vi "Spec Edit.vi"(4 "0기준?":bool, 5 "Condition":string[][](table), 6 "열번호(기준값)":i32, 7 "Spec Value":string[][](table), 8 "에러 입력(에러 없음)":errorcluster, 9 "Resolution":string[][](array[string]), 10 "Spec Default":string[][](table), 11 "Func_ext":string) -> (0 "에러 출력":errorcluster, 1 "변경?":bool, 2 "Spec Default out":string[][](array[string]), 3 "Spec 출력":string[][](array[string]))   [LabVIEW 2020]
uses:
  Controls/Cmd_Spec Edit.ctl
  Controls/Cmd_Mouse Popup.ctl
  Controls/Cmd_Var Data IO.ctl
  Variables/Global_Cal Info.vi
  Public/Polymorph/Cell Space_Table.vi
panel:
  in  "추가 단위":string
  in  "추가SPEC":string
  in  "적용":bool
  in  "초기화":bool
  in  "Default 단위":string
  in  "일괄변경":bool
  in  "하한":bool
  in  "상한":bool
  in  "상한하한":bool
  in  "스크롤 막대":i32(c297)
  in  "Default 값":string
  in  "취소":bool
  in  "확인":bool
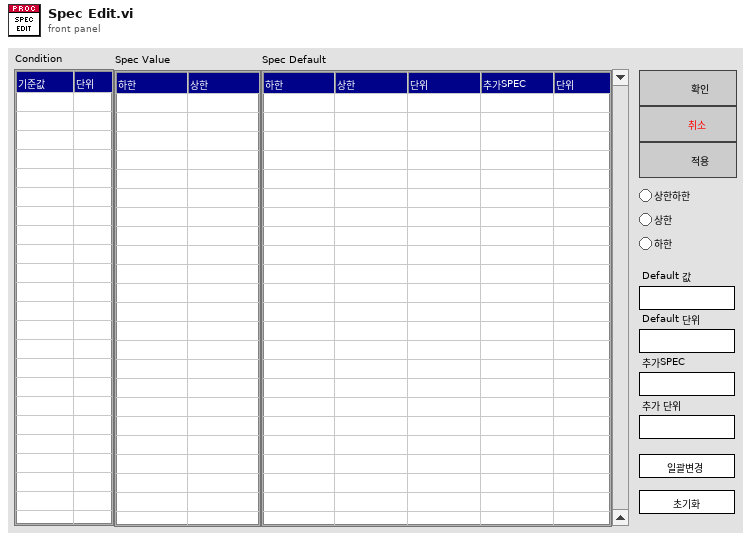
[diagram p1: front panel]
types:
  T1 = typedef "Cmd_Spec Edit.ctl" = enum16{"종료", "Start", "스펙계산", "이벤트대기"}
  T2 = typedef "Cmd_Mouse Popup.ctl" = enum16{"활성화", "메뉴선택"}
  T3 = typedef "Cmd_Var Data IO.ctl" = enum16{"Condition", "Condition Default", "Condition_Temp", "Resolution", "Resolution Default", "Resolution Old", "Spec", "Spec Default", "Spec Old", "Spec Temp", "Result", "Result2", "Result3", "Result_Temp", "Result_ADJ", "Result_ADJ2", "STD1", "STD2", "STD3", "STD4", "STD5", "STD Temp", "CMC", "CMC Default"}
  T4 = typedef "LVRectTypeDef.ctl" = cluster{"Left":i16, "Top":i16, "Right":i16, "Bottom":i16}
  T5 = cluster{"Shift":bool, "Ctrl":bool, "Alt":bool, "Cmd":bool, "Opt":bool}
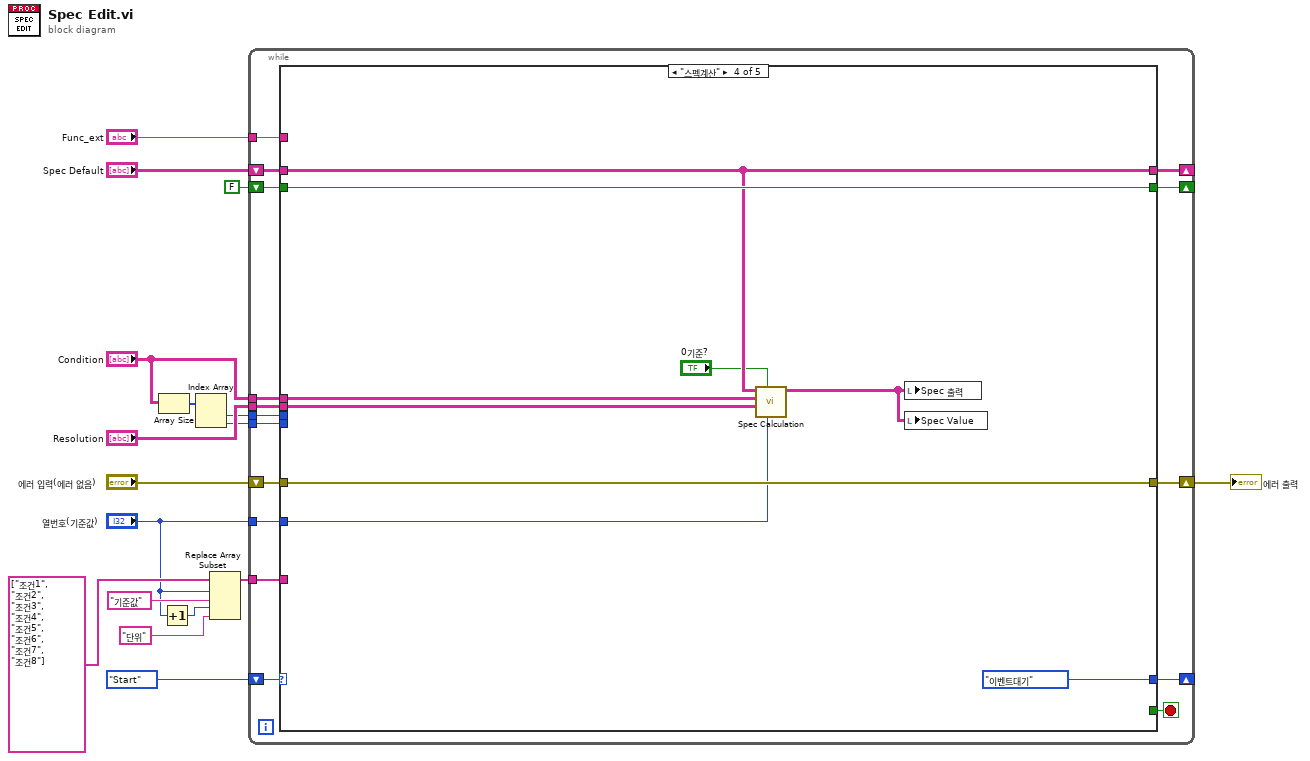
[diagram p0: block diagram]
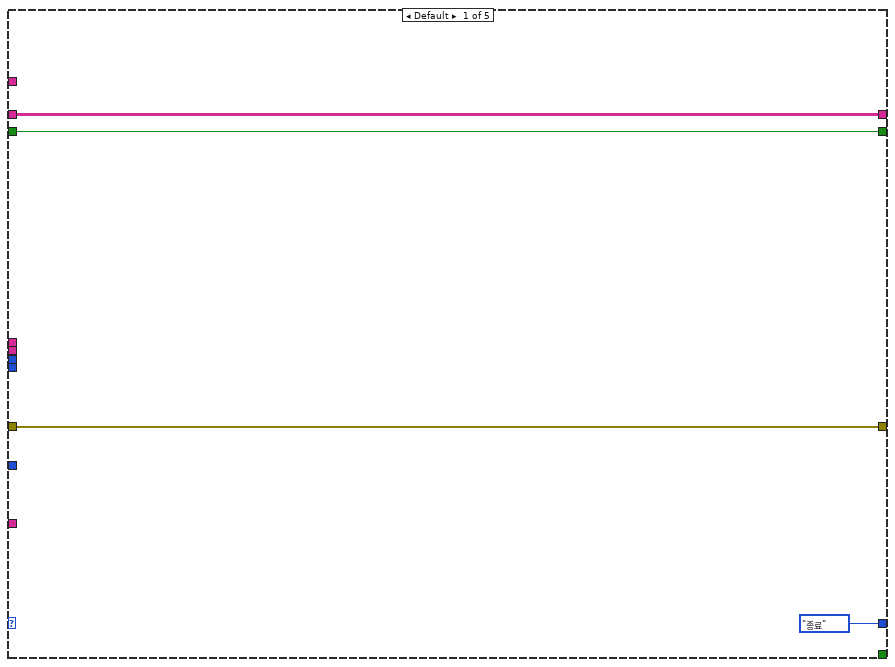
[diagram p2: hidden frame]
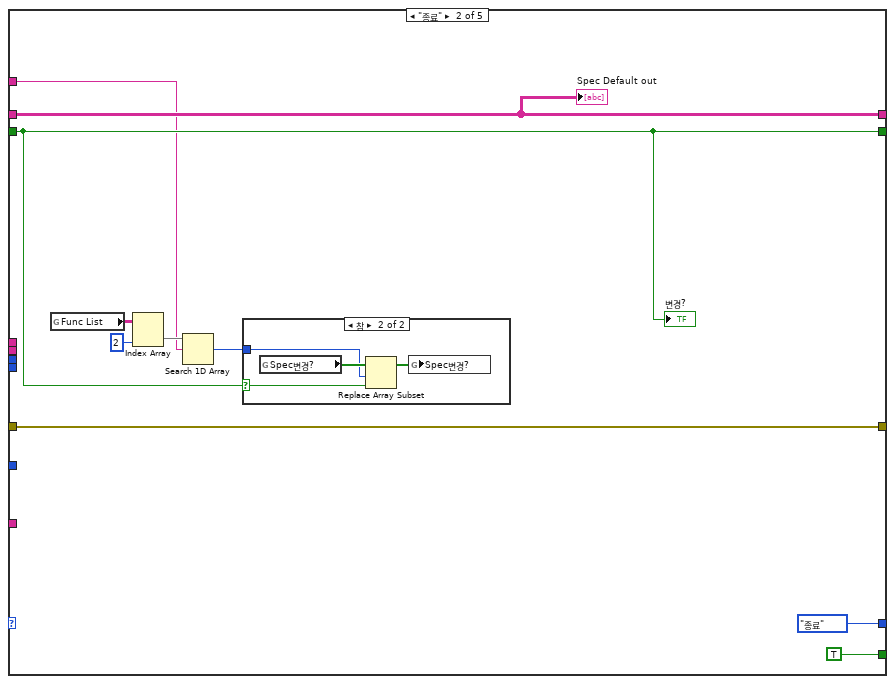
[diagram p3: hidden frame]
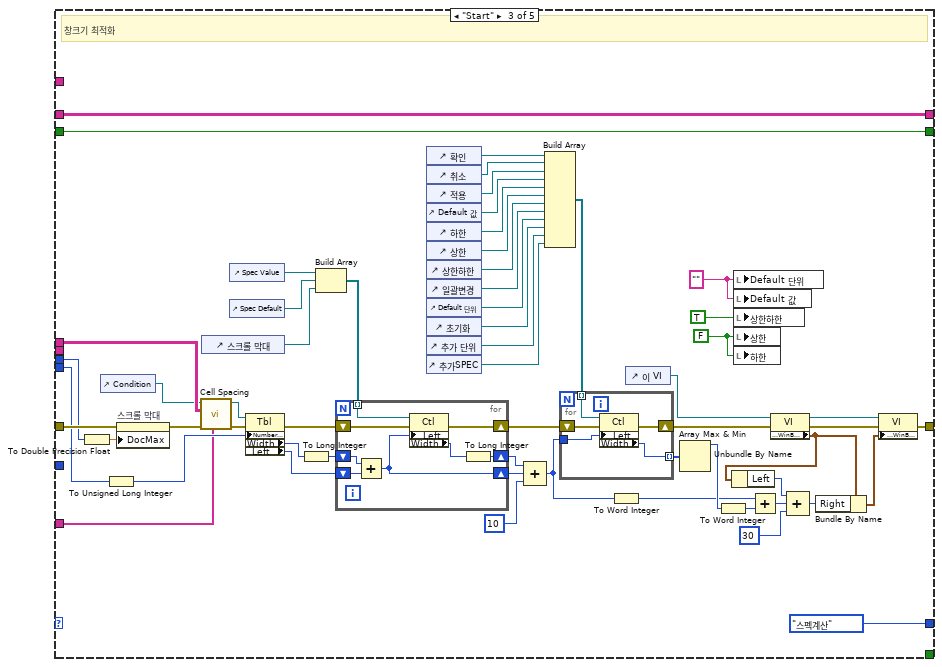
[diagram p5: hidden frame]
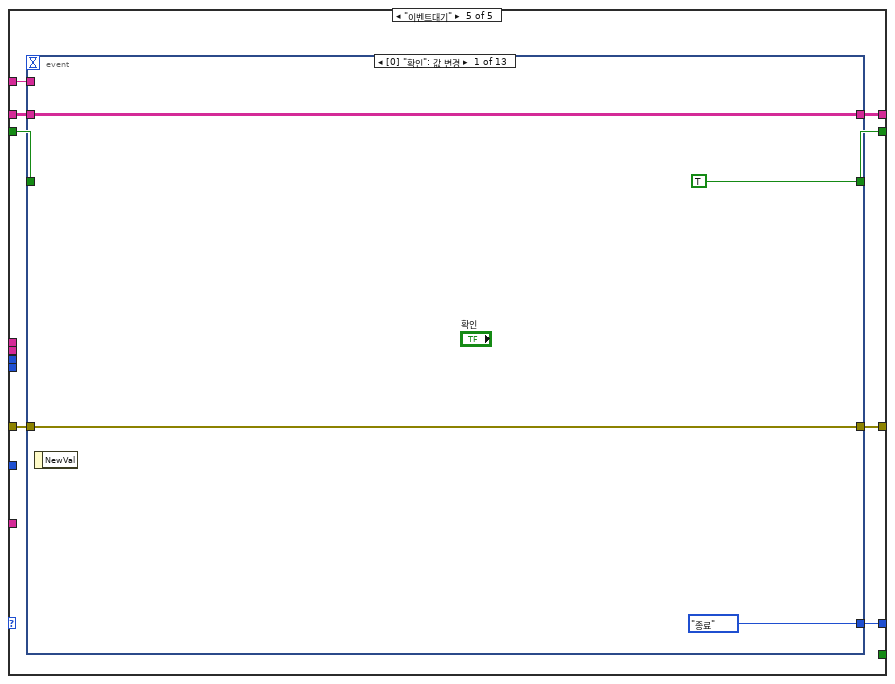
[diagram p6: hidden frame]
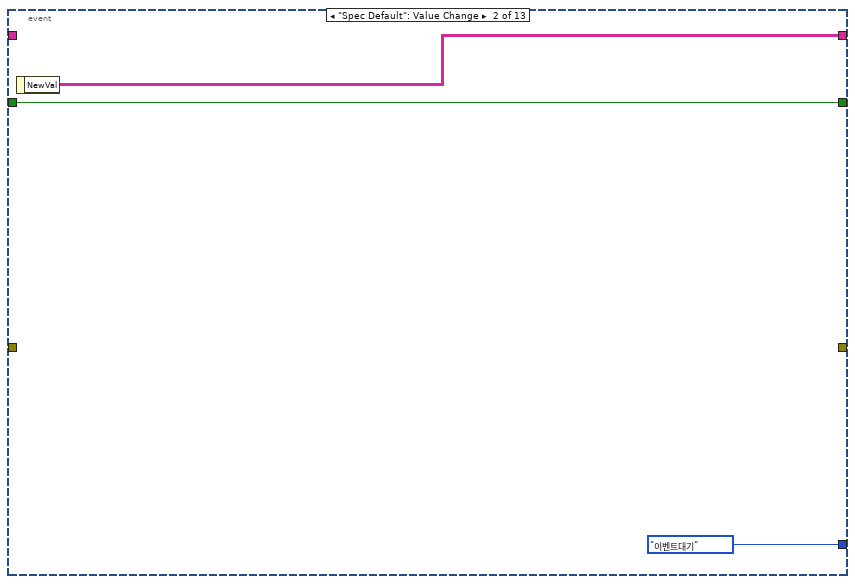
[diagram p7: hidden frame]
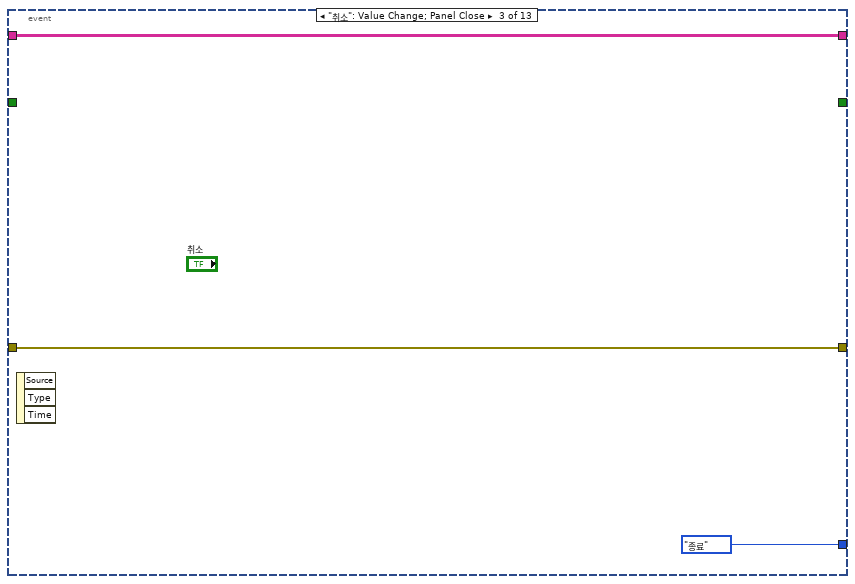
[diagram p8: hidden frame]
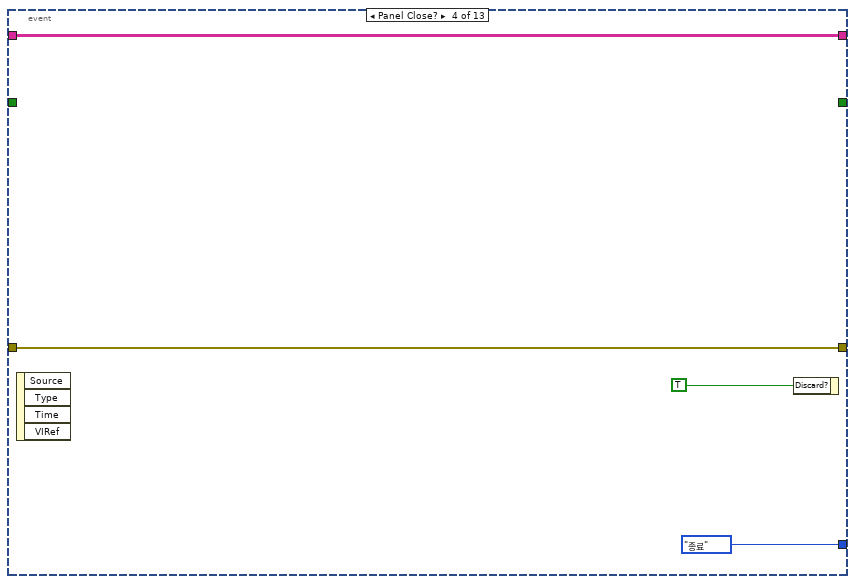
[diagram p9: hidden frame]
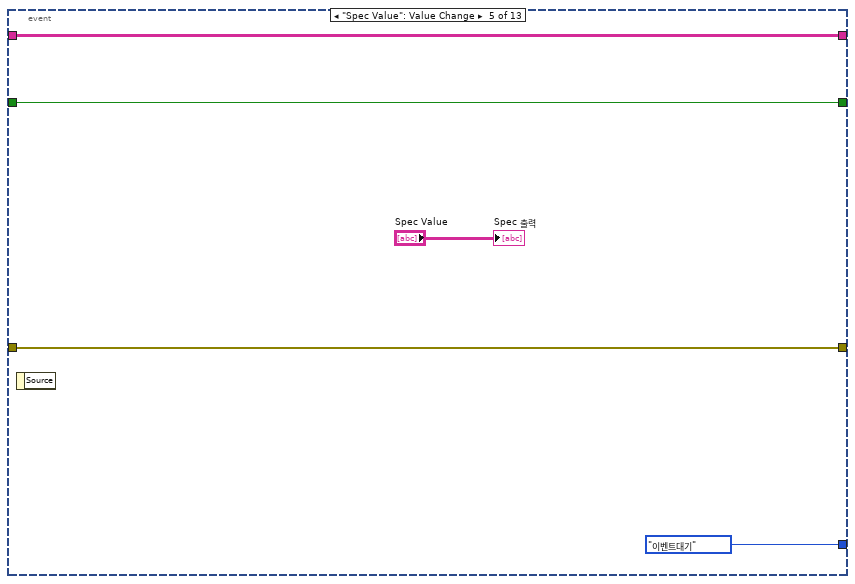
[diagram p10: hidden frame]
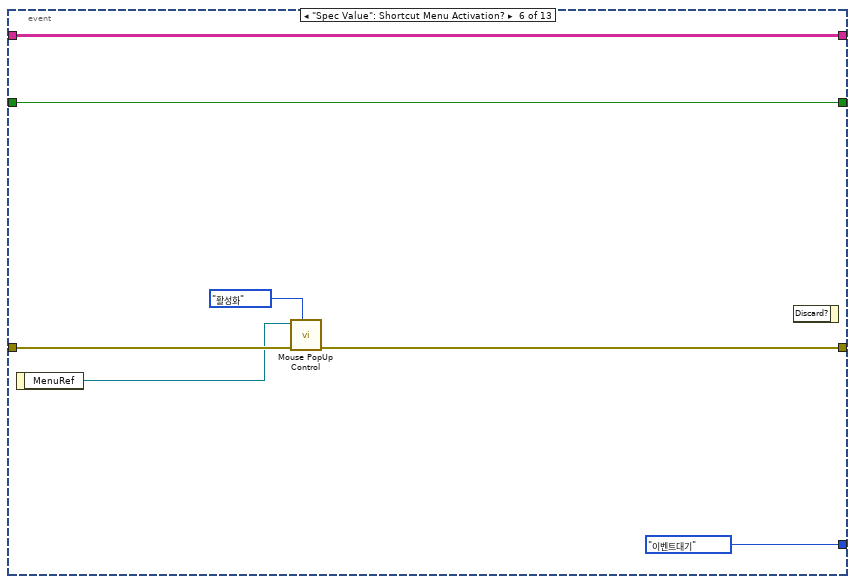
[diagram p11: hidden frame]
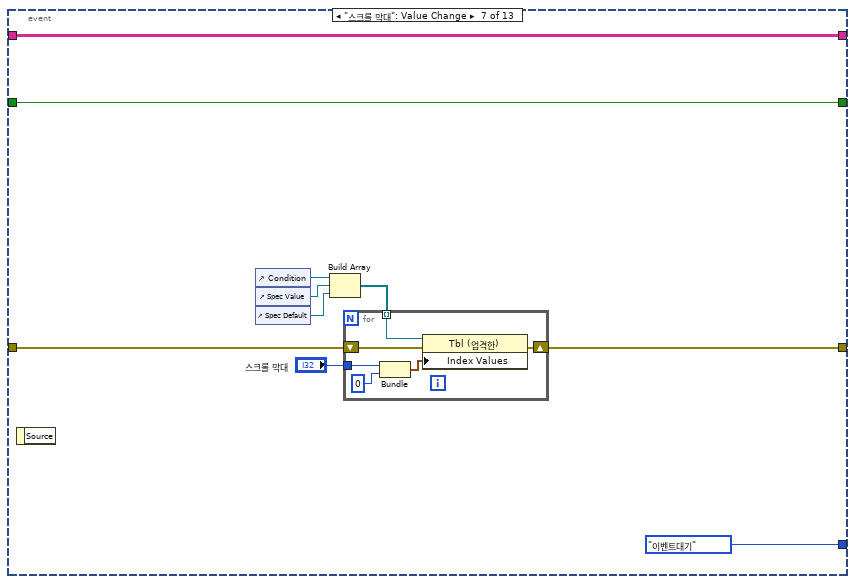
[diagram p12: hidden frame]
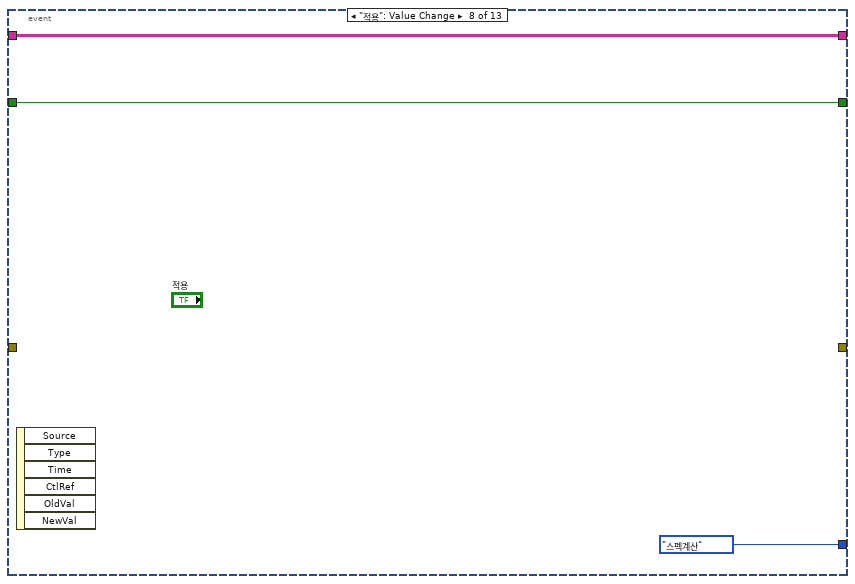
[diagram p13: hidden frame]
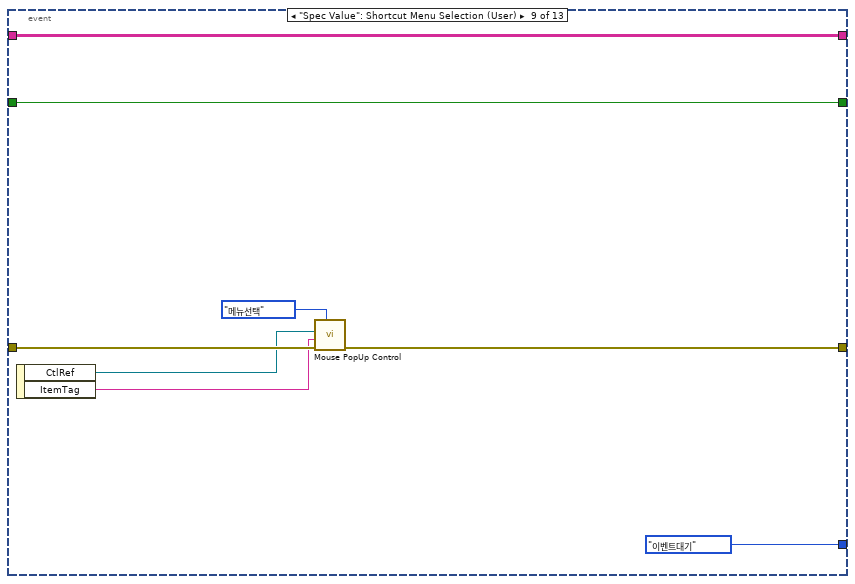
[diagram p14: hidden frame]
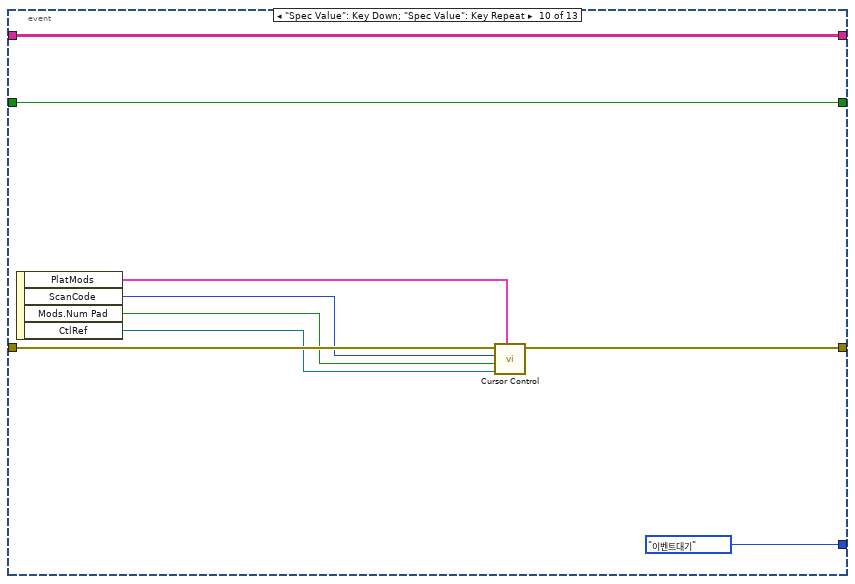
[diagram p15: hidden frame]
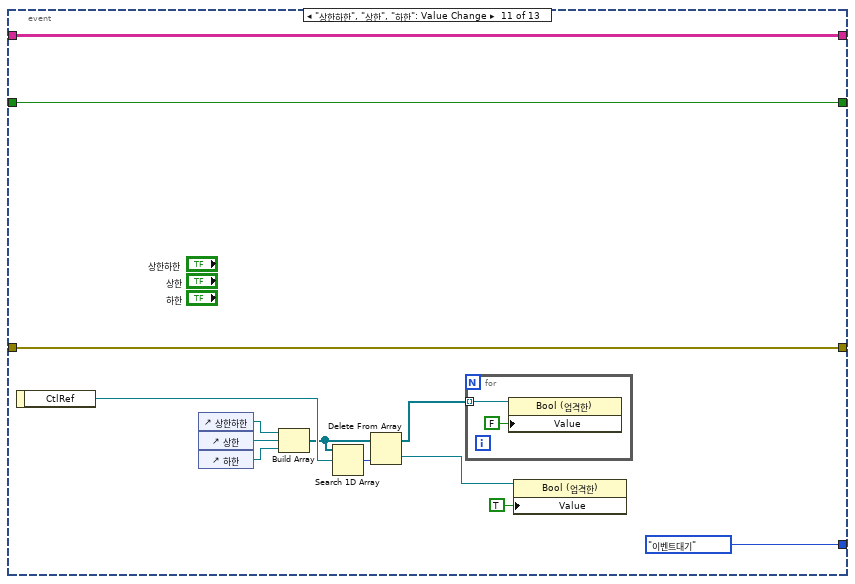
[diagram p16: hidden frame]
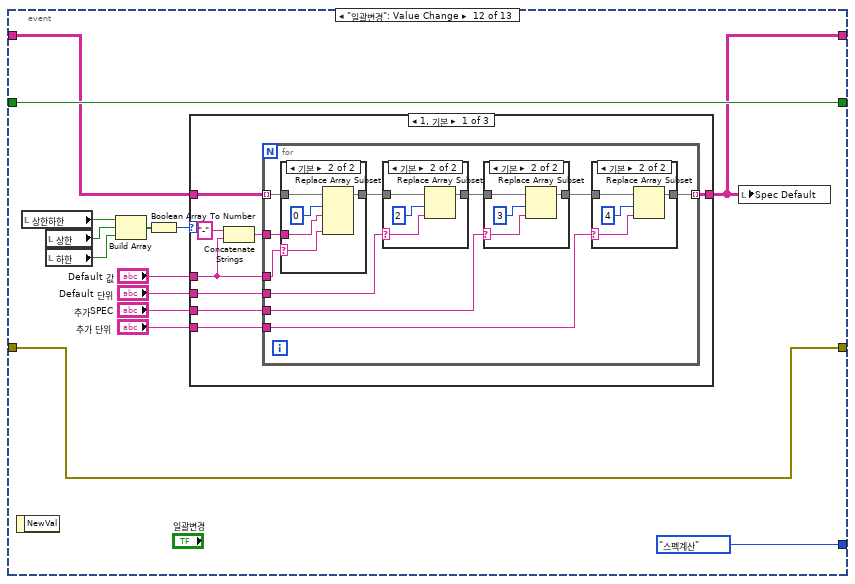
[diagram p17: hidden frame]
diagram:
  n1 = Array Size(array="Condition") -> (size(s)=w11:i32[])
  n2 = Increment(x="열번호(기준값)") -> (x+1=w1:i32)
  n3 = Index Array(array=w11) -> (element #1=w10:i32, element #2=w8:i32)  [unwired: 2 in]
  n4 = Replace Array Subset(array=string[] ["조건1", "조건2", "조건3", "조건4", "조건5", "조건6", "조건7", "조건8"] ("열 헤더 문자열[]"), new element #1="기준값" ("새 원소/부분배열"), index #1="열번호(기준값)", new element #2="단위" ("새 원소/부분배열"), index #2=w1) -> (w3:string[])
  n5 = while {
    tunnel: "Condition" -> [w31]
    shift-right: [w33] -> w15
    shift-left: "에러 입력(에러 없음)" -> [w32]
    shift-right: [w29] -> _
    shift-left: Cmd_Spec_Edit."Start" -> [w30]
    tunnel: "열번호(기준값)" -> [w28]
    shift-right: [w27] -> _
    shift-left: "Spec Default" -> [w26]
    shift-right: [w24] -> _
    shift-left: FALSE -> [w23]
    tunnel: "Resolution" -> [w22]
    tunnel: "Func_ext" -> [w21]
    tunnel: w10 -> [w20]
    tunnel: w8 -> [w19]
    tunnel: w3 -> [w18]
    stop <- w25 stop-if-true
    n6 = case shown="\"스펙계산\"" w30 {
      tunnel: [w37 w45 w86 w131 w138] -> w33
      tunnel: w32 -> [w37 w45 w71 w131 w139]
      tunnel: w31 -> [_ _ w60 w126 _]
      tunnel: [Cmd_Spec_Edit."종료" Cmd_Spec_Edit."종료" Cmd_Spec_Edit."스펙계산" Cmd_Spec_Edit."이벤트대기" w137] -> w29
      tunnel: w28 -> [_ _ _ w125 _]
      tunnel: [w35 w44 w83 w128 w135] -> w27
      tunnel: w26 -> [w35 w44 w83 w128 w136]
      tunnel: [_ TRUE _ _ _] -> w25
      tunnel: [w34 w43 w80 w129 w134] -> w24
      tunnel: w23 -> [w34 w43 w80 w129 w133]
      tunnel: w22 -> [_ _ _ w124 _]
      tunnel: w21 -> [_ w38 _ _ w132]
      tunnel: w20 -> [_ _ w70 _ _]
      tunnel: w19 -> [_ _ w69 _ _]
      tunnel: w18 -> [_ _ w61 _ _]
      frame Default {
      }
      frame "종료" {
        n7 = global read "Global_Cal Info.vi" "Func List"() -> (w40:string[][])
        n8 = Index Array(array=w40, index (col)=2 ("비활성화된 인덱스 (열)")) -> (element=w42:string[])  [unwired: 1 in]
        n9 = Search 1D Array(1D array=w42, element=w38) -> (index of element=w39:i32)  [unwired: 1 in]
        n10 = case shown="참" w43 {
          selector: w43 -> [_ w49]
          tunnel: w39 -> [_ w48]
          frame False {
          }
          frame True {
            n11 = global read "Global_Cal Info.vi" "Spec변경?"() -> (w51:bool[])
            n12 = Replace Array Subset(array=w51, new element=w49, index=w48) -> (w50:bool[])
            n13 = global write "Global_Cal Info.vi" "Spec변경?"(w50) -> ()
          }
        }
        "Spec Default out" <- w44
        "변경?" <- w43
      }
      frame "Start" {
        w72 = FALSE ("상한")
        w74 = "" ("Default 단위")
        # "창크기 최적화"
        n14 = To Double Precision Float(number=w70) -> (double precision float=w85:dbl)
        n15 = control-ref of="Condition"() -> (w58:refnum<vi>)
        n16 = To Unsigned Long Integer(number=w69) -> (unsigned 32bit integer=w87:u32)
        n17 = property on="스크롤 막대" class="Scroll (엄격한)"(error in=w71, "DocMax"=w85) -> (error out=w56:errorcluster)  [unwired: 1 in, 1 out]
        n18 = call-poly "Cell Spacing.vi"("Col Header in"=w61, "error in"=w56, "Data in"=w60, "테이블 참조 in"=w58) -> ("error out"=w55:errorcluster, "테이블 참조 Out"=w57:refnum<vi>)  [unwired: 5 in, 1 out]
        n19 = control-ref of="스크롤 막대"() -> (w88:refnum<vi>)
        n20 = control-ref of="Spec Value"() -> (w109:refnum<vi>)
        n21 = control-ref of="Spec Default"() -> (w108:refnum<vi>)
        n22 = property on="프로퍼티 노드" class="Tbl"(reference=w57, error in=w55, "Number of Columns"=w87) -> (error out=w59:errorcluster, "Width"=w68:u32, "Left"=w106:i32)  [unwired: 1 out]
        n23 = To Long Integer(number=w68) -> (32bit integer=w67:i32)
        n24 = Build Array(w109, w108, w88) -> (w107:refnum<vi>[])
        n25 = for {
          tunnel: w107 -> [w122] mode=indexing
          shift-right: [w117] -> w95
          shift-left: w67 -> [w115]
          shift-right: [w120] -> w94
          shift-left: w106 -> [w121]
          shift-right: [w118] -> w103
          shift-left: w59 -> [w119]
          n26 = Add(x=w115, y=w121) -> (x+y=w120:i32)
          n27 = property class="Ctl"(reference=w122, error in=w119, "Left"=w120) -> (error out=w118:errorcluster, "Width"=w116:u32)  [unwired: 1 out]
          n28 = To Long Integer(number=w116) -> (32bit integer=w117:i32)
        }
        n29 = control-ref of="확인"() -> (w102:refnum<vi>)
        n30 = control-ref of="취소"() -> (w101:refnum<vi>)
        n31 = control-ref of="적용"() -> (w54:refnum<vi>)
        n32 = control-ref of="Default 값"() -> (w100:refnum<vi>)
        n33 = control-ref of="하한"() -> (w79:refnum<vi>)
        n34 = control-ref of="상한"() -> (w78:refnum<vi>)
        n35 = control-ref of="상한하한"() -> (w77:refnum<vi>)
        n36 = control-ref of="일괄변경"() -> (w76:refnum<vi>)
        n37 = control-ref of="Default 단위"() -> (w75:refnum<vi>)
        n38 = control-ref of="초기화"() -> (w62:refnum<vi>)
        n39 = control-ref of="추가 단위"() -> (w53:refnum<vi>)
        n40 = control-ref of="추가SPEC"() -> (w52:refnum<vi>)
        n41 = Compound Arithmetic op=ADD(w95, w94, 10 ("y")) -> (w97:i32)
        n42 = Build Array(w102, w101, w54, w100, w79, w78, w77, w76, w75, w62, w53, w52) -> (w99:refnum<vi>[])
        n43 = for {
          shift-right: [w113] -> w66
          shift-left: w103 -> [w114]
          tunnel: w99 -> [w112] mode=indexing
          tunnel: w97 -> [w111]
          tunnel: [w110] -> w98 mode=indexing
          n44 = property class="Ctl"(reference=w112, error in=w114, "Left"=w111) -> (error out=w113:errorcluster, "Width"=w110:u32)  [unwired: 1 out]
        }
        n45 = To Word Integer(number=w97) -> (16bit integer=w81:i16)
        n46 = control-ref of="이 VI"() -> (w105:refnum<vi>)
        n47 = Array Max & Min(array=w98) -> (max value=w96:u32)  [unwired: 3 out]
        n48 = To Word Integer(number=w96) -> (16bit integer=w65:i16)
        n49 = local write "Default 단위"(w74) -> ()
        n50 = local write "Default 값"(w74) -> ()
        n51 = local write "상한하한"(TRUE ("상한하한")) -> ()
        n52 = local write "상한"(w72) -> ()
        n53 = local write "하한"(w72) -> ()
        n54 = Add(x=w81, y=w65) -> (x+y=w82:i16)
        n55 = property class="VI"(reference=w105, error in=w66) -> (reference out=w104:refnum<vi>, error out=w63:errorcluster, "Front Panel.WinBounds"=w91:T4)
        n56 = Unbundle By Name(w91) -> ("Left"=w90:i16)
        n57 = Compound Arithmetic op=ADD(w90, w82, i16 30 ("y")) -> (w64:i16)
        n58 = Bundle By Name(cluster=w91, "Right"=w64) -> (w89:T4)
        n59 = property class="VI"(reference=w104, error in=w63, "Front Panel.WinBounds"=w89) -> (error out=w86:errorcluster)  [unwired: 1 out]
      }
      frame "스펙계산" {
        n60 = call "Spec Calculation.vi"("기준값 열번호"=w125, "0기준?"="0기준?", "Resolution"=w124, "Condition in"=w126, "Spec Default"=w128) -> ("Spec out"=w127:string[][])  [unwired: 5 in, 1 out]
        n61 = local write "Spec 출력"(w127) -> ()
        n62 = local write "Spec Value"(w127) -> ()
      }
      frame "이벤트대기" {
        n63 = event shown="[0] \"확인\": 값 변경" {
          selector: _ -> [_ _ _ _ _ _ _ _ _ _ _ _ _]
          dyn-events: _ -> [_ _ _ _ _ _ _ _ _ _ _ _ _]
          timeout: _ -> [_ _ _ _ _ _ _ _ _ _ _ _ _]
          tunnel: w139 -> [w143 _ w149 w150 w158 w165 w172 _ w192 w201 w211 w229 w298]
          tunnel: [w143 _ w149 w150 w158 w164 w171 _ w191 w200 w211 w229 w295] -> w138
          tunnel: [Cmd_Spec_Edit."종료" Cmd_Spec_Edit."이벤트대기" Cmd_Spec_Edit."종료" Cmd_Spec_Edit."종료" Cmd_Spec_Edit."이벤트대기" Cmd_Spec_Edit."이벤트대기" Cmd_Spec_Edit."이벤트대기" Cmd_Spec_Edit."스펙계산" Cmd_Spec_Edit."이벤트대기" Cmd_Spec_Edit."이벤트대기" Cmd_Spec_Edit."이벤트대기" Cmd_Spec_Edit."스펙계산" Cmd_Spec_Edit."스펙계산"] -> w137
          tunnel: w136 -> [w141 _ w147 w151 w155 w161 w168 w184 w187 w196 w214 w220 _]
          tunnel: [w141 w145 w147 w151 w155 w161 w168 w184 w187 w196 w214 w219 w294] -> w135
          tunnel: [TRUE w146 _ _ w156 w160 w167 w183 w186 w195 w213 w230 w300] -> w134
          tunnel: w133 -> [_ w146 _ _ w156 w160 w167 w183 w186 w195 w213 w230 w300]
          tunnel: w132 -> [_ _ _ _ _ _ _ _ _ _ _ _ w297]
          event "확인": Value Change {
            n64 = event-data() -> ()  [unwired: 1 in, 1 out]
          }
          event "Spec Default": Value Change {
            n65 = event-data() -> ("NewVal"=w145:string[][])  [unwired: 1 in]
          }
          event "취소": Value Change; Panel Close {
            n66 = event-data() -> ()  [unwired: 1 in, 3 out]
          }
          event Panel Close? {
            n67 = event-data() -> ()  [unwired: 1 in, 4 out]
            n68 = event-data("Discard?"=TRUE ("버림?")) -> ()  [unwired: 1 in, 1 out]
          }
          event "Spec Value": Value Change {
            n69 = event-data() -> ()  [unwired: 1 in, 1 out]
            "Spec 출력" <- "Spec Value"
          }
          event "Spec Value": Shortcut Menu Activation? {
            n70 = event-data() -> ("MenuRef"=w162:refnum<k9>)  [unwired: 1 in]
            n71 = call "Mouse PopUp Control.vi"("type"=Cmd_Mouse_Popup."활성화", "error in"=w165, "메뉴 참조"=w162) -> ("error out"=w164:errorcluster)  [unwired: 8 in]
            n72 = event-data() -> ()  [unwired: 2 in, 1 out]
          }
          event "스크롤 막대": Value Change {
            n73 = event-data() -> ()  [unwired: 1 in, 1 out]
            n74 = control-ref of="Condition"() -> (w175:refnum<vi>)
            n75 = control-ref of="Spec Value"() -> (w174:refnum<vi>)
            n76 = control-ref of="Spec Default"() -> (w173:refnum<vi>)
            n77 = Build Array(w175, w174, w173) -> (w170:refnum<vi>[])
            n78 = for {
              tunnel: w170 -> [w179] mode=indexing
              shift-right: [w180] -> w171
              shift-left: w172 -> [w181]
              tunnel: "스크롤 막대" -> [w178]
              n79 = Bundle("스크롤 막대"=w178, 0) -> (w177:cluster{"스크롤 막대":i32, i32})  [unwired: 1 in]
              n80 = property class="Tbl (엄격한)"(reference=w179, error in=w181, "Index Values"=w177) -> (error out=w180:errorcluster)  [unwired: 1 out]
            }
          }
          event "적용": Value Change {
            n81 = event-data() -> ()  [unwired: 1 in, 6 out]
          }
          event "Spec Value": Shortcut Menu Selection (User) {
            n82 = event-data() -> ("CtlRef"=w189:refnum<vi>, "ItemTag"=w188:string)  [unwired: 1 in]
            n83 = call "Mouse PopUp Control.vi"("type"=Cmd_Mouse_Popup."메뉴선택", "error in"=w192, "아이템 태그"=w188, "Tbl 참조 번호"=w189) -> ("error out"=w191:errorcluster)  [unwired: 7 in]
          }
          event "Spec Value": Key Down; "Spec Value": Key Repeat {
            n84 = event-data() -> ("PlatMods"=w193:T5, "ScanCode"=w199:i16, "Mods.Num Pad"=w198:bool, "CtlRef"=w197:refnum<vi>)  [unwired: 1 in]
            n85 = call "Cursor Control.vi"("플랫폼 조합키"=w193, "참조"=w197, "Num Pad"=w198, "ScanCode"=w199, "error in"=w201) -> ("error out"=w200:errorcluster)  [unwired: 5 in, 1 out]
          }
          event "상한하한", "상한", "하한": Value Change {
            n86 = event-data() -> ("CtlRef"=w207:refnum<vi>)  [unwired: 1 in]
            n87 = control-ref of="상한하한"() -> (w210:refnum<vi>)
            n88 = control-ref of="상한"() -> (w209:refnum<vi>)
            n89 = control-ref of="하한"() -> (w208:refnum<vi>)
            n90 = Build Array(w210, w209, w208) -> (w206:refnum<vi>[])
            n91 = Search 1D Array(1D array=w206, element=w207) -> (index of element=w205:i32)  [unwired: 1 in]
            n92 = Delete From Array(array=w206, index=w205) -> (deleted portion=w203:refnum<vi>, array with subset deleted=w204:refnum<vi>[])  [unwired: 1 in]
            n93 = for {
              tunnel: w204 -> [w216] mode=indexing
              n94 = property class="Bool (엄격한)"(reference=w216, "Value"=FALSE ("값")) -> ()  [unwired: 1 in, 2 out]
            }
            n95 = property class="Bool (엄격한)"(reference=w203, "Value"=TRUE ("값")) -> ()  [unwired: 1 in, 2 out]
          }
          event "일괄변경": Value Change {
            n96 = event-data() -> ()  [unwired: 1 in, 1 out]
            n97 = local read "상한하한"() -> (w227:bool)
            n98 = local read "상한"() -> (w226:bool)
            n99 = local read "하한"() -> (w225:bool)
            n100 = Build Array(w227, w226, w225) -> (w224:bool[])
            n101 = Boolean Array To Number(Boolean array=w224) -> (number=w223:u32)
            n102 = case shown="1, 기본" w223 {
              tunnel: "Default 값" -> [w235 w270 w283]
              tunnel: w220 -> [w237 w274 w285]
              tunnel: "Default 단위" -> [w234 w271 w282]
              tunnel: [w231 w273 w284] -> w219
              tunnel: "추가SPEC" -> [w233 _ _]
              tunnel: "추가 단위" -> [w232 _ _]
              frame 1, Default {
                n103 = Concatenate Strings("-" ("문자열"), w235) -> (w236:string)
                n104 = for {
                  tunnel: w237 -> [w239] mode=indexing
                  tunnel: w236 -> [w240]
                  tunnel: w235 -> [w248]
                  tunnel: w234 -> [w247]
                  tunnel: w233 -> [w244]
                  tunnel: w232 -> [w243]
                  tunnel: [w241] -> w231 mode=indexing
                  n105 = case shown="기본" w248 {
                    selector: w248 -> [_ w267]
                    tunnel: w239 -> [w264 w269]
                    tunnel: [w264 w268] -> w246
                    tunnel: w240 -> [_ w265]
                    frame "" {
                    }
                    frame Default {
                      n106 = Replace Array Subset(array=w269, new element #1=w265, index #1=0, new element #2=w267) -> (w268:string[])  [unwired: 1 in]
                    }
                  }
                  n107 = case shown="기본" w247 {
                    selector: w247 -> [_ w260]
                    tunnel: w246 -> [w259 w263]
                    tunnel: [w259 w262] -> w245
                    frame "" {
                    }
                    frame Default {
                      n108 = Replace Array Subset(array=w263, new element=w260, index=2) -> (w262:string[])
                    }
                  }
                  n109 = case shown="기본" w244 {
                    selector: w244 -> [_ w255]
                    tunnel: w245 -> [w254 w258]
                    tunnel: [w254 w257] -> w242
                    frame "" {
                    }
                    frame Default {
                      n110 = Replace Array Subset(array=w258, new element=w255, index=3) -> (w257:string[])
                    }
                  }
                  n111 = case shown="기본" w243 {
                    selector: w243 -> [_ w250]
                    tunnel: w242 -> [w249 w253]
                    tunnel: [w249 w252] -> w241
                    frame "" {
                    }
                    frame Default {
                      n112 = Replace Array Subset(array=w253, new element=w250, index=4) -> (w252:string[])
                    }
                  }
                }
              }
              frame 2 {
                n113 = for {
                  tunnel: w274 -> [w281] mode=indexing
                  tunnel: 1 -> [w280]
                  tunnel: w270 -> [w278]
                  tunnel: [w277] -> w273 mode=indexing
                  tunnel: w271 -> [w275]
                  n114 = Replace Array Subset(array=w281, new element=w278, index=w280) -> (w279:string[])
                  n115 = Replace Array Subset(array=w279, new element=w275, index=2 ("인덱스")) -> (w277:string[])
                }
              }
              frame 4 {
                n116 = for {
                  tunnel: w285 -> [w293] mode=indexing
                  tunnel: 0 -> [w292]
                  tunnel: w283 -> [w290]
                  tunnel: [w289] -> w284 mode=indexing
                  tunnel: w282 -> [w287]
                  n117 = Replace Array Subset(array=w293, new element=w290, index=w292) -> (w291:string[])
                  n118 = Replace Array Subset(array=w291, new element=w287, index=2 ("인덱스")) -> (w289:string[])
                }
              }
            }
            n119 = local write "Spec Default"(w219) -> ()
          }
          event "초기화": Value Change {
            n120 = event-data() -> ()  [unwired: 1 in, 1 out]
            n121 = call "Variables Data IO.vi"("Select"=Cmd_Var_Data_IO."Spec Default", "error in"=w298, "Func_ext"=w297) -> ("error out"=w295:errorcluster, "Data Out"=w294:string[][])  [unwired: 6 in, 1 out]
            n122 = local write "Spec Default"(w294) -> ()
          }
        }
      }
    }
  }
  "에러 출력" <- w15
